vi "线性转换.vi"(7 "AD0":dbl, 8 "转换值最大值":dbl, 9 "转换值最小值":dbl, 10 "原始值最大值":dbl, 11 "原始值最小值":dbl) -> (3 "数值":dbl)   [LabVIEW 2016, in "环境动力监测库.lvlib"]
uses:
  <vilib>/Analysis/6fits.llb/Curve Fitting Criteria.ctl
  <vilib>/Analysis/NI_AALPro.lvlib
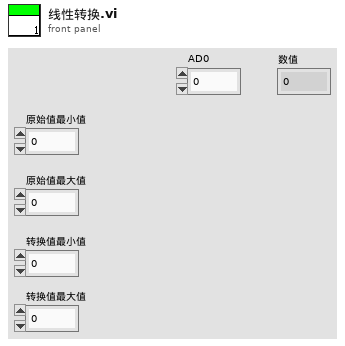
[diagram p1: front panel]
types:
  T1 = typedef "NI_AALPro.lvlib/Curve Fitting Criteria.ctl" = u16
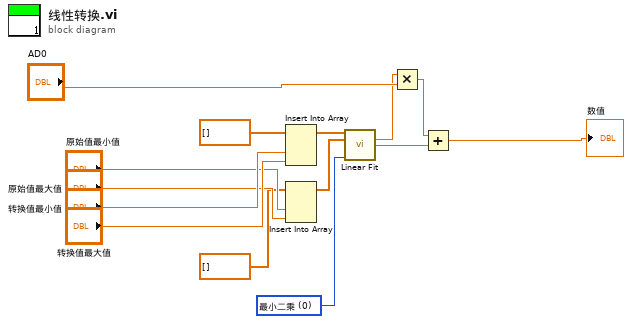
[diagram p0: block diagram]
diagram:
  w1 = T1 0 items=["最小二乘", "最小绝对残差", "Bisquare"] ("method")
  n1 = Insert Into Array(array=dbl[] [] ("数组"), new element #1="转换值最小值", new element #2="转换值最大值") -> (w9:dbl[])  [unwired: 1 in]
  n2 = Insert Into Array(array=dbl[] [] ("数组"), new element #1="原始值最小值", new element #2="原始值最大值") -> (w8:dbl[])  [unwired: 1 in]
  n3 = call <vilib>:"Linear Fit.vi"("Y"=w9, "X"=w8, "method"=w1) -> ("slope"=w10:dbl, "intercept"=w13:dbl)  [unwired: 8 in, 3 out]
  n4 = Multiply(x=w10, y="AD0") -> (x*y=w12:dbl)
  n5 = Add(x=w12, y=w13) -> (x+y=→"数值":dbl)
